vi "ApplyRules.vi"(11 "Numeric":u64) -> (2 "StoneSplit":bool, 3 "Array":u64[](array[numeric]))   [LabVIEW 2023, in "2024_11.lvclass"]
uses:
  2024_11.lvclass
  2024_11.lvclass/2024_11.ctl
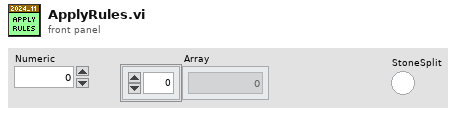
[diagram p1: front panel]
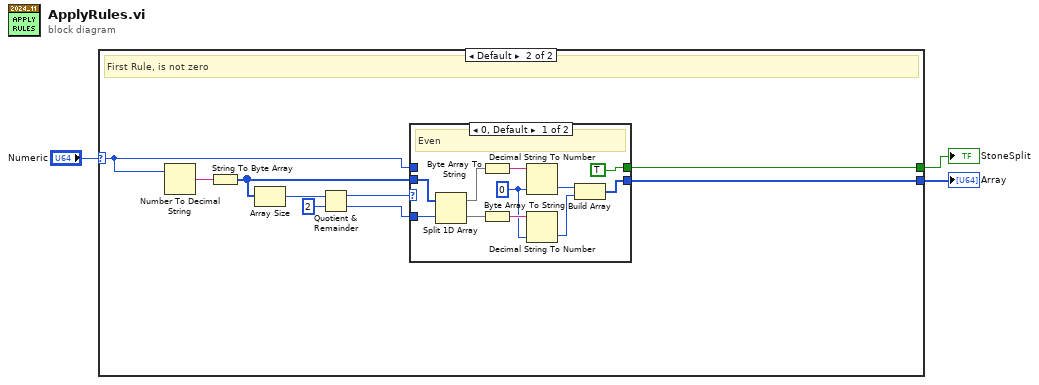
[diagram p0: block diagram]
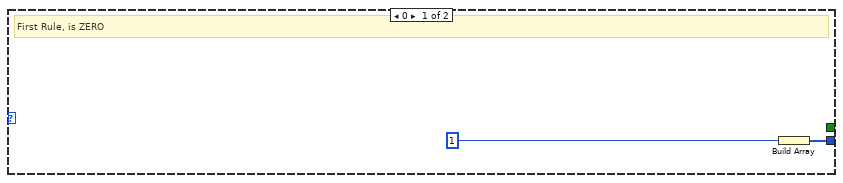
[diagram p2: hidden frame]
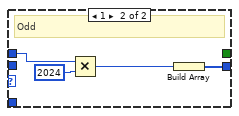
[diagram p3: hidden frame]
diagram:
  n1 = case shown="Default" "Numeric" {
    selector: "Numeric" -> [_ w13]
    tunnel: [w5 w14] -> w2
    tunnel: [_ w12] -> w1
    frame 0 {
      # "First Rule, is ZERO"
      n2 = Build Array(u64 1) -> (w5:u64[])
    }
    frame Default {
      # "First Rule, is not zero"
      n3 = Number To Decimal String(number=w13) -> (decimal integer string=w11:string)  [unwired: 1 in]
      n4 = String To Byte Array(string=w11) -> (unsigned byte array=w7:u8[])
      n5 = Array Size(array=w7) -> (size(s)=w10:i32)
      n6 = Quotient & Remainder(x=w10, y=2) -> (x-y*floor(x/y)=w8:i32, floor(x/y)=w6:i32)
      n7 = case shown="0, Default" w8 {
        tunnel: w7 -> [w25 _]
        tunnel: w6 -> [w24 _]
        tunnel: [w19 w27] -> w14
        tunnel: w13 -> [_ w29]
        tunnel: [TRUE _] -> w12
        frame 0, Default {
          w18 = u64 0
          # "Even"
          n8 = Split 1D Array(array=w25, index=w24) -> (first subarray=w23:u8[], second subarray=w22:u8[])
          n9 = Byte Array To String(unsigned byte array=w23) -> (string=w20:string)
          n10 = Byte Array To String(unsigned byte array=w22) -> (string=w21:string)
          n11 = Decimal String To Number(string=w20, default (0L)=w18) -> (number=w17:u64)  [unwired: 1 in, 1 out]
          n12 = Decimal String To Number(string=w21, default (0L)=w18) -> (number=w16:u64)  [unwired: 1 in, 1 out]
          n13 = Build Array(w17, w16) -> (w19:u64[])
        }
        frame 1 {
          # "Odd"
          n14 = Multiply(x=w29, y=u64 2024) -> (x*y=w26:u64)
          n15 = Build Array(w26) -> (w27:u64[])
        }
      }
    }
  }
  "Array" <- w2
  "StoneSplit" <- w1
